vi "HovaCAL_Interface_SetPumpRun.vi"(8 "error in (no error)":errorcluster caption="Fehler (Eingang, kein Fehler)", 9 "sofort":bool=TRUE, 11 "run":bool) -> (0 "error out":errorcluster caption="Fehler (Ausgang)")   [LabVIEW 2020, in "Linearisierung v2.lvlib" / "Gasteiler.lvlib" / "HovaCAL_Interface.lvlib" / "Kommunikation.lvlib"]
uses:
  Kommunikation.lvlib
  Aktion_FGV_HovaCAL_Interface_SetData.ctl
  Aktion_FGV_HovaCAL_Interface_Kommunikation.ctl
  Aktion_FGV_HovaCAL_Interface_Kommandos.ctl
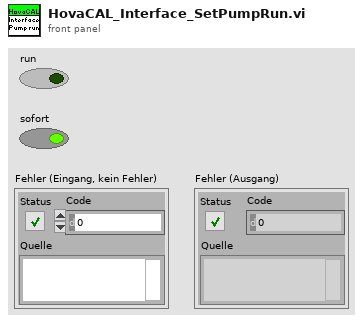
[diagram p1: front panel]
types:
  T1 = typedef "Linearisierung v2.lvlib/Gasteiler.lvlib/HovaCAL_Interface.lvlib/Kommunikation.lvlib/Aktion_FGV_HovaCAL_Interface_SetData.ctl" = enum16{"lesen", "Konzentrationen", "Pumpen Parameter", "Pumpe Konzentration", "Pumpe run", "Temperaturen", "Fluss", "Limits", "init"}
  T2 = typedef "Linearisierung v2.lvlib/Gasteiler.lvlib/HovaCAL_Interface.lvlib/Controls.lvlib/Pump Dry Mode.ctl" = i32
  T3 = typedef "Linearisierung v2.lvlib/Gasteiler.lvlib/HovaCAL_Interface.lvlib/Controls.lvlib/Pump Control Mode.ctl" = u32
  T4 = cluster{"running?":bool, "dry mode":T2, "control mode":T3}
  T5 = typedef "Linearisierung v2.lvlib/Gasteiler.lvlib/HovaCAL_Interface.lvlib/Kommunikation.lvlib/Aktion_FGV_HovaCAL_Interface_Kommandos.ctl" = enum16{"lesen", "verarbeiten", "hinzufügen", "on top", "init", "sammeln", "freigeben", "connected"}
  T6 = typedef "Linearisierung v2.lvlib/Gasteiler.lvlib/HovaCAL_Interface.lvlib/Kommunikation.lvlib/Aktion_FGV_HovaCAL_Interface_Kommunikation.ctl" = enum16{"Initialisieren", "Set Konzentrationen", "Set Gase", "Set Limits", "Get Dynamische Werte", "Beenden", "Com ändern", "Get Gase init", "Pause", "Get Gasteiler Infos", "Get MFC Infos", "Set Pumpen Parameter", "Set Pumpe Konzenration", "Set Pumpe run", "Set Temperaturen", "Set Fluss", "Get Gase", "Get Limits", "Get Dynamische Werte 1", "Get Dynamische Werte 2"}
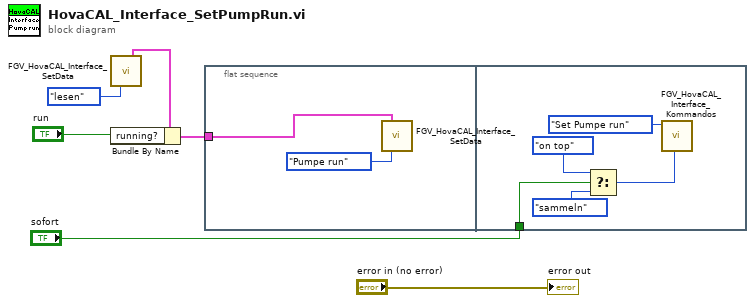
[diagram p0: block diagram]
diagram:
  n1 = call "FGV_HovaCAL_Interface_SetData.vi"("Aktion"=Aktion_FGV_HovaCAL_Interface_SetData."lesen") -> ("PumpModeGeneral-Cluster out"=w3:T4)  [unwired: 8 in, 6 out]
  n2 = Bundle By Name(cluster=w3, "running?"="run") -> (w5:T4)
  n3 = flat-sequence {
    tunnel: w5 -> [w7]
    tunnel: "sofort" -> [w9]
    frame #0 {
      n4 = call "FGV_HovaCAL_Interface_SetData.vi"("PumpModeGeneral-Cluster in"=w7, "Aktion"=Aktion_FGV_HovaCAL_Interface_SetData."Pumpe run") -> ()  [unwired: 7 in, 7 out]
    }
    frame #1 {
      n5 = Select(t=Aktion_FGV_HovaCAL_Interface_Kommandos."on top" ("Aktion"), s=w9, f=Aktion_FGV_HovaCAL_Interface_Kommandos."sammeln") -> (s? t:f=w10:T5)
      n6 = call "FGV_HovaCAL_Interface_Kommandos.vi"("Aktion"=w10, "Kommando in"=Aktion_FGV_HovaCAL_Interface_Kommunikation."Set Pumpe run") -> ()  [unwired: 3 in, 6 out]
    }
  }
  "error out" <- "error in (no error)"
